vi "Remove Controls from Selection.vi"(8 "Error In":errorcluster, 11 "Selection":refnum<vi>[](array[refnum])) -> (0 "Error Out":errorcluster, 3 "Filtered Selection":refnum<vi>[](array[refnum]))   [LabVIEW 2017, in "Eulogy.lvlib"]
uses:
  Eulogy.lvlib
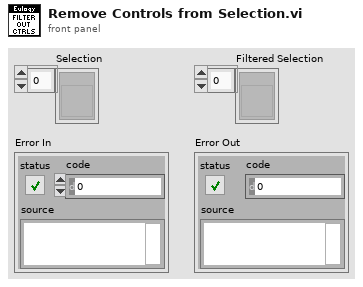
[diagram p1: front panel]
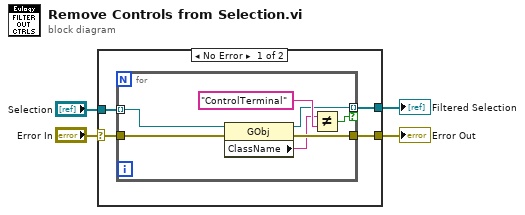
[diagram p0: block diagram]
diagram:
  n1 = case shown="No Error" "Error In" {
    selector: "Error In" -> [w5 w16]
    tunnel: [w8 w17] -> w4
    tunnel: [w7 w16] -> w3
    tunnel: "Selection" -> [w6 w17]
    frame No Error {
      n2 = for {
        tunnel: w6 -> [w14] mode=indexing
        tunnel: [w11] -> w8 mode=indexing if=w10
        tunnel: w5 -> [w13]
        tunnel: [w12] -> w7
        n3 = property class="GObj"(reference=w14, error in=w13) -> (reference out=w11:refnum<vi>, error out=w12:errorcluster, "ClassName"=w9:string)
        n4 = Not Equal?(x=w9, y="ControlTerminal") -> (x != y?=w10:bool)
      }
    }
    frame Error {
    }
  }
  "Filtered Selection" <- w4
  "Error Out" <- w3
